vi "ID_Connection.vi"(11 "error in":errorcluster) -> (4 "Arduino":refnum<visa-resource-name>, 6 "Arduino":bool, 8 "Pump":refnum<visa-resource-name>, 10 "Pump":bool, 15 "error out":errorcluster)   [LabVIEW 2019]
uses:
  <vilib>/Instr/_visa.llb/VISA Find Search Mode.ctl
  <vilib>/Instr/_visa.llb/VISA Configure Serial Port (Instr).vi
  <vilib>/regexp/Match Regular Expression.xnode
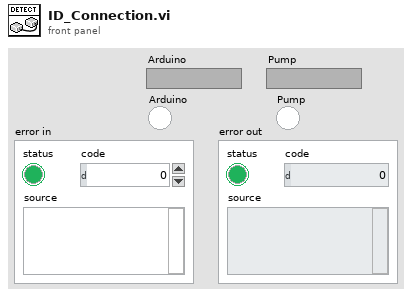
[diagram p1: front panel]
types:
  T1 = typedef "VISA Find Search Mode.ctl" = u32
  T2 = cluster{"VISA resource name":refnum<visa-resource-name>, "error out":errorcluster}
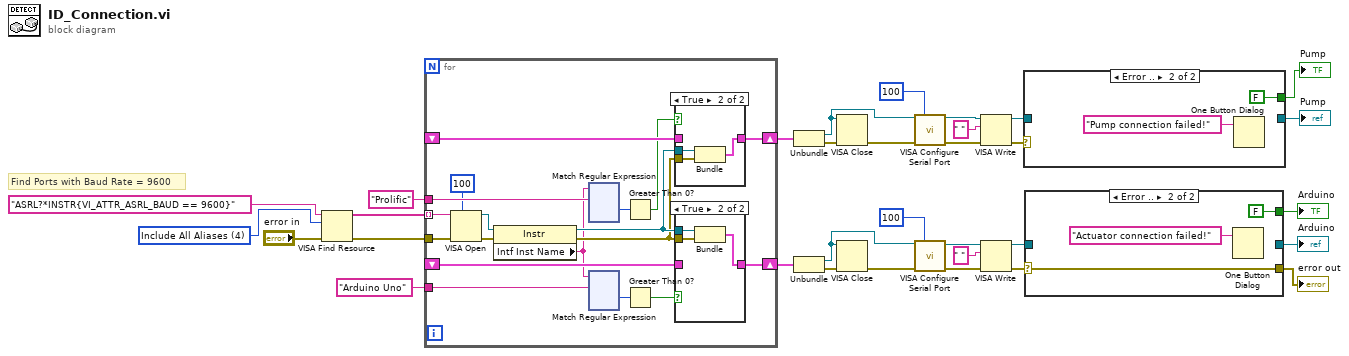
[diagram p0: block diagram]
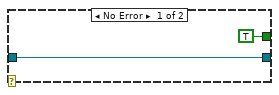
[diagram p2: hidden frame]
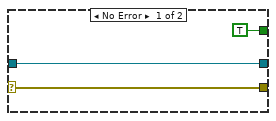
[diagram p3: hidden frame]
diagram:
  w20 = T1 4 items=["Canonical Names Only"=0, "Aliases Only"=2, "Include Matching Aliases"=3, "Include All Aliases"=4] ("Search Mode")
  # "Find Ports with Baud Rate = 9600"
  n1 = VISA Find Resource(8:"error in", 10:w20, 11:"ASRL?*INSTR{VI_ATTR_ASRL_BAUD == 9600}" ("expression (\"?*\")")) -> (0:w29:errorcluster, 3:w32:string[])  [unwired: 1 out]
  n2 = for {
    tunnel: w32 -> [w50] mode=indexing
    tunnel: "Arduino Uno" -> [w46]
    shift-right: [w44] -> w31
    shift-left: _ -> [w43]
    tunnel: w29 -> [w42]
    shift-right: [w41] -> w13
    shift-left: _ -> [w40]
    tunnel: "Prolific" -> [w35]
    n3 = VISA Open(timeout (0)=u32 100 ("VISA Open timeout (0)"), error in (no error)=w42, VISA resource name=w50) -> (VISA resource name=w49:refnum<visa-resource-name>, error out=w45:errorcluster)  [unwired: 2 in]
    n4 = property class="Instr"(reference=w49, error in=w45) -> (reference out=w37:refnum<visa-resource-name>, error out=w36:errorcluster, "Intf Inst Name"=w34:string)
    n5 = xnode "Match Regular Expression"("input string"=w34, "regular expression"=w35) -> ("offset past match"=w39:i32)  [unwired: 4 in, 4 out]
    n6 = xnode "Match Regular Expression"("input string"=w34, "regular expression"=w46) -> ("offset past match"=w48:i32)  [unwired: 4 in, 4 out]
    n7 = Greater Than 0?(x=w39) -> (x > 0?=w38:bool)
    n8 = Greater Than 0?(x=w48) -> (x > 0?=w47:bool)
    n9 = case shown="True" w38 {
      tunnel: w37 -> [_ w168]
      tunnel: w36 -> [_ w167]
      tunnel: [w165 w166] -> w41
      tunnel: w40 -> [w165 _]
      frame False {
      }
      frame True {
        n10 = Bundle("VISA resource name"=w168, "error out"=w167) -> (w166:T2)  [unwired: 1 in]
      }
    }
    n11 = case shown="True" w47 {
      tunnel: w37 -> [_ w172]
      tunnel: w36 -> [_ w171]
      tunnel: [w169 w170] -> w44
      tunnel: w43 -> [w169 _]
      frame False {
      }
      frame True {
        n12 = Bundle("VISA resource name"=w172, "error out"=w171) -> (w170:T2)  [unwired: 1 in]
      }
    }
  }
  n13 = Unbundle(w13) -> ("VISA resource name"=w11:refnum<visa-resource-name>, "error out"=w12:errorcluster)
  n14 = Unbundle(w31) -> ("VISA resource name"=w21:refnum<visa-resource-name>, "error out"=w26:errorcluster)
  n15 = VISA Close(VISA resource name=w11, error in (no error)=w12) -> (error out=w17:errorcluster)
  n16 = VISA Close(VISA resource name=w21, error in (no error)=w26) -> (error out=w25:errorcluster)
  n17 = call-poly "VISA Configure Serial Port"("VISA resource name"=w11, "timeout (10sec)"=u32 100, "error in (no error)"=w17) -> ("VISA resource name out"=w16:refnum<visa-resource-name>, "error out"=w15:errorcluster)  [unwired: 11 in]
  n18 = call-poly "VISA Configure Serial Port"("VISA resource name"=w21, "timeout (10sec)"=u32 100, "error in (no error)"=w25) -> ("VISA resource name out"=w24:refnum<visa-resource-name>, "error out"=w23:errorcluster)  [unwired: 11 in]
  n19 = VISA Write(VISA resource name=w16, write buffer=" ", error in (no error)=w15) -> (VISA resource name out=w3:refnum<visa-resource-name>, error out=w5:errorcluster)  [unwired: 1 out]
  n20 = VISA Write(VISA resource name=w24, write buffer=" ", error in (no error)=w23) -> (VISA resource name out=w10:refnum<visa-resource-name>, error out=w9:errorcluster)  [unwired: 1 out]
  n21 = case shown="Error .." w5 {
    tunnel: [w288 _] -> w4
    tunnel: w3 -> [w288 _]
    tunnel: [TRUE FALSE] -> w2
    frame No Error {
    }
    frame Error {
      n22 = One Button Dialog(message="Pump connection failed!") -> ()  [unwired: 1 in, 1 out]
    }
  }
  "Pump" <- w4
  "Pump" <- w2
  n23 = case shown="Error .." w9 {
    selector: w9 -> [w291 w295]
    tunnel: [TRUE FALSE] -> w6
    tunnel: w10 -> [w292 _]
    tunnel: [w292 _] -> w7
    tunnel: [w291 w295] -> w8
    frame No Error {
    }
    frame Error {
      n24 = One Button Dialog(message="Actuator connection failed!") -> ()  [unwired: 1 in, 1 out]
    }
  }
  "Arduino" <- w7
  "error out" <- w8
  "Arduino" <- w6
